vi "CheckAndCheckmate.vi"(2 "Castling State":bool[][](array[boolean]), 3 "Black/White Turn (T/F)":bool, 4 "Board":i32[][](array[numeric])=[[-3, -5, -4, -2, -1, -4, -5, -3], [-6, -6, -6, -6, -6, -6, -6, -6], [0, 0, 0, 0, 0, 0, 0, 0], [0, 0, 0, 0, 0, 0, 0, 0], [0, 0, 0, 0, 0, 0, 0, 0], [0, 0, 0, 0, 0, 0, 0, 0], [6, 6, 6, 6, 6, 6, 6, 6], [3, 5, 4, 2, 1, 4, 5, 3]]) -> (0 "Check":bool, 1 "Checkmate":bool)   [LabVIEW 2014]
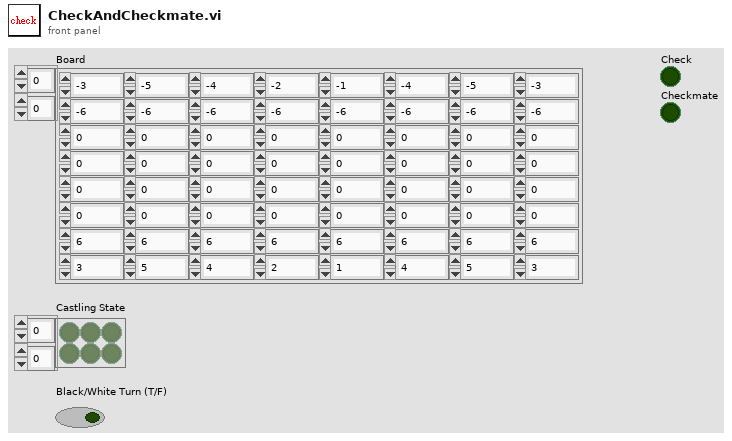
[diagram p1: front panel]
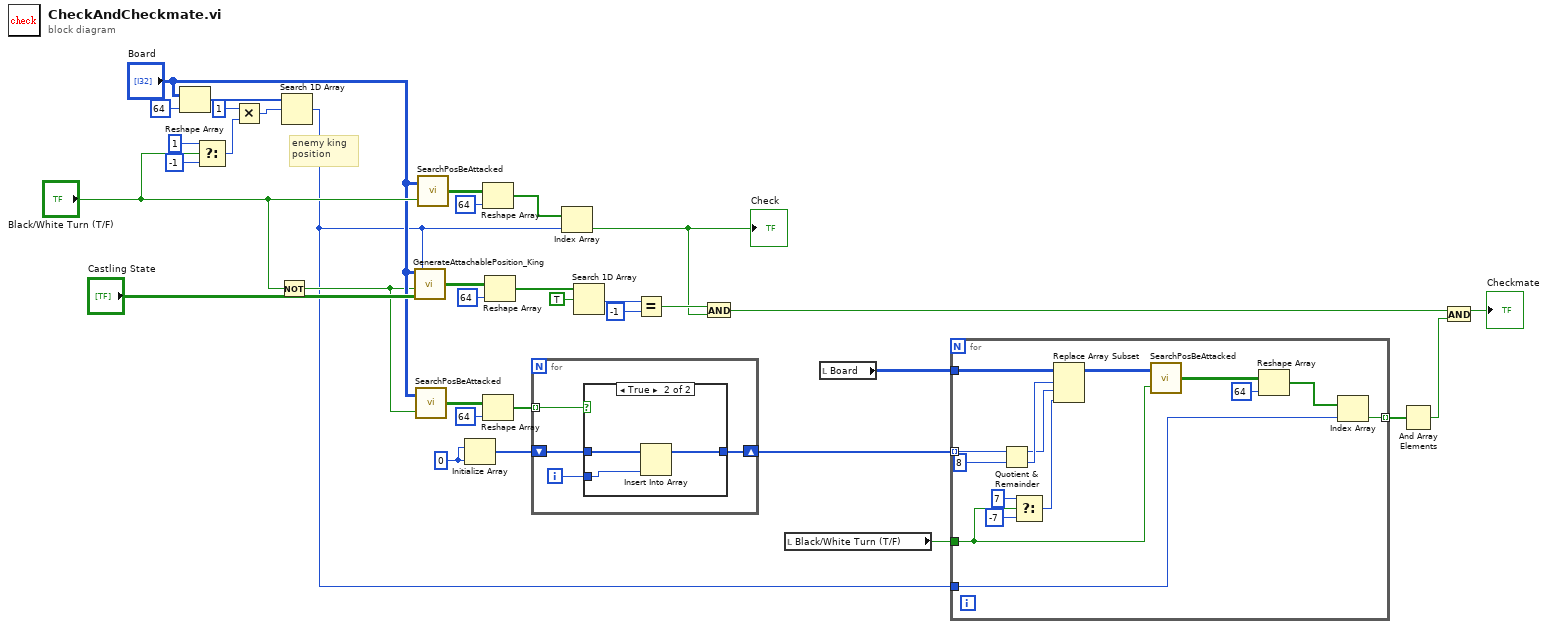
[diagram p0: block diagram]
diagram:
  w8 = 0 ("dimension size")
  # "enemy king\nposition"
  n1 = Reshape Array("Board", 64 ("dimension size")) -> (w34:i32[])
  n2 = Select(t=1, s="Black/White Turn (T/F)", f=-1) -> (s? t:f=w31:i32)
  n3 = Multiply(x=1, y=w31) -> (x*y=w32:i32)
  n4 = Not(x="Black/White Turn (T/F)") -> (.not. x?=w13:bool)
  n5 = Search 1D Array(1D array=w34, element=w32) -> (index of element=w4:i32)  [unwired: 1 in]
  n6 = call "GenerateAttachablePosition_King.vi"("Castling State"="Castling State", "Black/White Turn (T/F)"=w13, "pieceIndex"=w4, "Board"="Board") -> ("AttachablePosition"=w23:bool[][])
  n7 = call "SearchPosBeAttacked.vi"("Black/White (T/F)"=w13, "Board"="Board") -> ("AttackablePosition"=w11:bool[][])
  n8 = call "SearchPosBeAttacked.vi"("Black/White (T/F)"="Black/White Turn (T/F)", "Board"="Board") -> ("AttackablePosition"=w26:bool[][])
  n9 = Initialize Array(w8, w8) -> (w9:i32[])
  n10 = Reshape Array(w26, 64 ("dimension size")) -> (w25:bool[])
  n11 = Reshape Array(w11, 64 ("dimension size")) -> (w10:bool[])
  n12 = Reshape Array(w23, 64 ("dimension size")) -> (w22:bool[])
  n13 = for {
    tunnel: w10 -> [w39] mode=indexing
    shift-right: [w37] -> w7
    shift-left: w9 -> [w36]
    i -> [w38]
    n14 = case shown="True" w39 {
      tunnel: w38 -> [_ w41]
      tunnel: [w40 w43] -> w37
      tunnel: w36 -> [w40 w42]
      frame False {
      }
      frame True {
        n15 = Insert Into Array(array=w42, new element=w41) -> (w43:i32[])  [unwired: 1 in]
      }
    }
  }
  n16 = Index Array(array=w25, index=w4) -> (element=w17:bool)
  "Check" <- w17
  n17 = Search 1D Array(1D array=w22, element=TRUE) -> (index of element=w20:i32)  [unwired: 1 in]
  n18 = Equal?(x=w20, y=-1) -> (x = y?=w18:bool)
  n19 = And(x=w18, y=w17) -> (x .and. y?=w16:bool)
  n20 = local read "Black/White Turn (T/F)"() -> (w5:bool)
  n21 = local read "Board"() -> (w6:i32[][])
  n22 = for {
    tunnel: w7 -> [w58] mode=indexing
    tunnel: w6 -> [w55]
    tunnel: w5 -> [w49]
    tunnel: w4 -> [w45]
    tunnel: [w44] -> w3 mode=indexing
    n23 = Quotient & Remainder(x=w58, y=8) -> (x-y*floor(x/y)=w54:i32, floor(x/y)=w56:i32)
    n24 = Select(t=7, s=w49, f=-7) -> (s? t:f=w53:i32)
    n25 = Replace Array Subset(array=w55, new element=w53, index (row)=w56, index (col)=w54) -> (w50:i32[][])
    n26 = call "SearchPosBeAttacked.vi"("Black/White (T/F)"=w49, "Board"=w50) -> ("AttackablePosition"=w46:bool[][])
    n27 = Reshape Array(w46, 64 ("dimension size")) -> (w47:bool[])
    n28 = Index Array(array=w47, index=w45) -> (element=w44:bool)
  }
  n29 = And Array Elements(Boolean array=w3) -> (logical AND=w1:bool)
  n30 = And(x=w16, y=w1) -> (x .and. y?=→"Checkmate":bool)
